vi "RSZVB Set UI Port Binary Data.vi"(8 "error in (no error)":errorcluster {"code" format="%.0x"}, 9 "Data (0)":i32, 10 "Port (1)":i32=1, 11 "VISA session":refnum<visa-resource-name>) -> (0 "error out":errorcluster {"code" format="%.0x"}, 3 "dup VISA session":refnum<visa-resource-name>)   [LabVIEW 2011]
doc: "Writes a 0 or 1 to the output ports (pin 3 or 4) of the Universal Interface connector. The port lines have negative logic: A \"0\" corresponds to a high signal, a \"1\" to a low signal.\n\nRemote-control command(s):\nCONTrol:HANDler:OUTPut<port>[:DATA]"
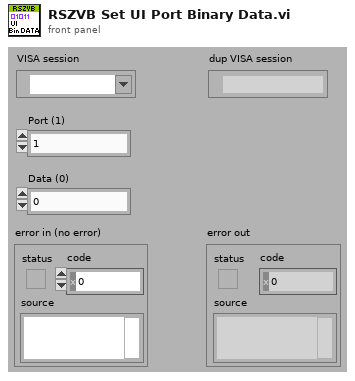
[diagram p1: front panel]
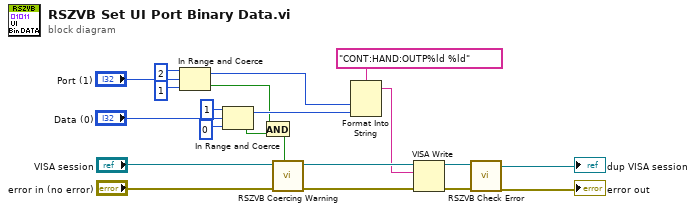
[diagram p0: block diagram]
diagram:
  n1 = In Range and Coerce(upper limit=2, x="Port (1)", lower limit=1) -> (coerced(x)=w1:i32, In Range?=w11:bool)
  n2 = In Range and Coerce(upper limit=1, x="Data (0)", lower limit=0) -> (coerced(x)=w12:i32, In Range?=w10:bool)
  n3 = And(x=w11, y=w10) -> (x .and. y?=w9:bool)
  n4 = call "RSZVB Coercing Warning.vi"("In Range?"=w9, "error in (no error)"="error in (no error)", "VISA session"="VISA session") -> ("error out"=w18:errorcluster, "dup VISA session"=w19:refnum<visa-resource-name>)  [unwired: 7 in]
  n5 = Format Into String(format string="CONT:HAND:OUTP%ld %ld", w1, w12) -> (resulting string=w15:string)  [unwired: 2 in, 1 out]
  n6 = VISA Write(VISA resource name=w19, write buffer=w15, error in (no error)=w18) -> (VISA resource name out=w16:refnum<visa-resource-name>, error out=w17:errorcluster)  [unwired: 1 out]
  n7 = call "RSZVB Check Error.vi"("error in (no error)"=w17, "VISA session"=w16) -> ("error out"=→"error out":errorcluster, "dup VISA session"=→"dup VISA session":refnum<visa-resource-name>)  [unwired: 8 in]
